vi "CRYMark Frame Above.vi"() -> ()   [LabVIEW 2013]
uses:
  <vilib>/Utility/miscctls.llb/LVPositionTypeDef.ctl
  SubVI/CRYMain Sub Window Global.vi
panel:
  in  "sMe":string
  in  "bShow":bool=TRUE
  in  "Above":bool
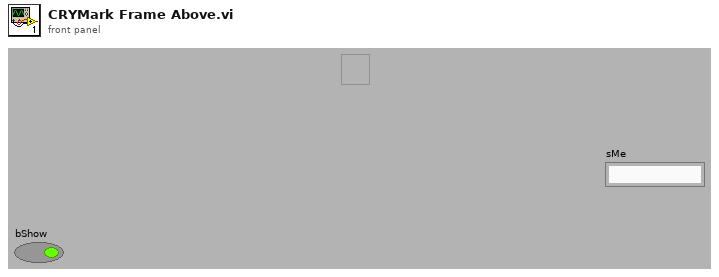
[diagram p1: front panel]
types:
  T1 = typedef "LVPositionTypeDef.ctl" = cluster{"Left":i32, "Top":i32}
  T2 = typedef "LVRectTypeDef.ctl" = cluster{"Left":i16, "Top":i16, "Right":i16, "Bottom":i16}
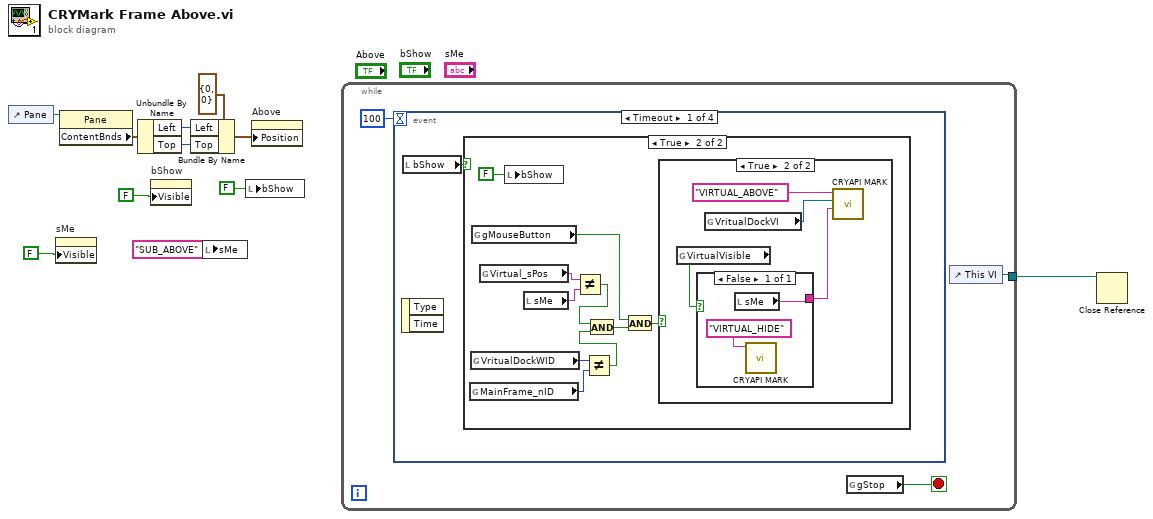
[diagram p0: block diagram]
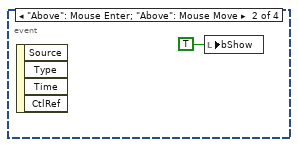
[diagram p4: hidden frame]
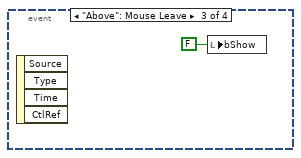
[diagram p5: hidden frame]
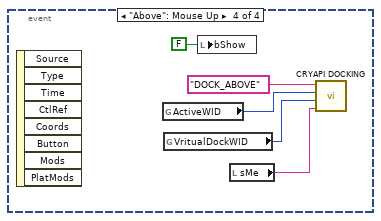
[diagram p6: hidden frame]
diagram:
  n1 = control-ref of="Pane"() -> (w11:refnum<vi>)
  n2 = property on="sMe" class="Str"("Visible"=FALSE) -> ()  [unwired: 2 in, 2 out]
  n3 = property class="Pane"(reference=w11) -> ("ContentBnds"=w10:T2)  [unwired: 1 in, 2 out]
  n4 = Unbundle By Name(w10) -> ("Left"=w9:i16, "Top"=w7:i16)
  n5 = property on="bShow" class="Bool (strict)"("Visible"=FALSE) -> ()  [unwired: 2 in, 2 out]
  n6 = Bundle By Name(cluster=T1 {"Left"=0, "Top"=0} ("Position"), "Left"=w9, "Top"=w7) -> (w6:T1)
  n7 = local write "sMe"("SUB_ABOVE" ("sMe")) -> ()
  n8 = local write "bShow"(FALSE ("bShow")) -> ()
  n9 = property on="Above" class="Bool (strict)"("Position"=w6) -> ()  [unwired: 2 in, 2 out]
  n10 = while {
    tunnel: [w12] -> w1
    stop <- w13 stop-if-true
    n11 = event shown="[0] Timeout" {
      selector: _ -> [_ _ _ _]
      dyn-events: _ -> [_ _ _ _]
      timeout: 100 -> [_ _ _ _]
      event Timeout {
        n12 = event-data() -> ()  [unwired: 3 out]
        n13 = local read "bShow"() -> (w15:bool)
        n14 = case shown="True" w15 {
          frame False {
          }
          frame True {
            n15 = global read "CRYMain Sub Window Global.vi" "MainFrame_nID"() -> (w24:i32)
            n16 = global read "CRYMain Sub Window Global.vi" "VritualDockWID"() -> (w23:i32)
            n17 = global read "CRYMain Sub Window Global.vi" "gMouseButton"() -> (w20:bool)
            n18 = global read "CRYMain Sub Window Global.vi" "Virtual_sPos"() -> (w19:string)
            n19 = local write "bShow"(FALSE ("bShow")) -> ()
            n20 = local read "sMe"() -> (w18:string)
            n21 = Not Equal?(x=w19, y=w18) -> (x != y?=w22:bool)
            n22 = Not Equal?(x=w23, y=w24) -> (x != y?=w16:bool)
            n23 = And(x=w22, y=w16) -> (x .and. y?=w21:bool)
            n24 = And(x=w20, y=w21) -> (x .and. y?=w25:bool)
            n25 = case shown="True" w25 {
              frame False {
              }
              frame True {
                n26 = global read "CRYMain Sub Window Global.vi" "VirtualVisible"() -> (w28:bool)
                n27 = case shown="False, True" w28 {
                  tunnel: [w30] -> w26
                  frame False {
                    n28 = local read "sMe"() -> (w30:string)
                    n29 = call "CRYAPI MARK.vi"("sAction"="VIRTUAL_HIDE") -> ()  [unwired: 3 in, 7 out]
                  }
                }
                n30 = global read "CRYMain Sub Window Global.vi" "VritualDockVI"() -> (w29:refnum<vi>)
                n31 = call "CRYAPI MARK.vi"("sAction"="VIRTUAL_ABOVE", "mVritual_VIRef"=w29, "sData"=w26) -> ()  [unwired: 1 in, 7 out]
              }
            }
          }
        }
      }
      event "Above": Mouse Enter; "Above": Mouse Move {
        n32 = event-data() -> ()  [unwired: 5 out]
        n33 = local write "bShow"(TRUE ("bShow")) -> ()
      }
      event "Above": Mouse Leave {
        n34 = event-data() -> ()  [unwired: 5 out]
        n35 = local write "bShow"(FALSE ("bShow")) -> ()
      }
      event "Above": Mouse Up {
        n36 = event-data() -> ()  [unwired: 9 out]
        n37 = global read "CRYMain Sub Window Global.vi" "ActiveWID"() -> (w37:i32)
        n38 = global read "CRYMain Sub Window Global.vi" "VritualDockWID"() -> (w35:i32)
        n39 = local write "bShow"(FALSE ("bShow")) -> ()
        n40 = local read "sMe"() -> (w34:string)
        n41 = call "CRYAPI DOCKING.vi"("sData"=w34, "nDWinID"=w35, "nSWinID"=w37, "sAction"="DOCK_ABOVE") -> ()  [unwired: 8 out]
      }
    }
    n42 = global read "CRYMain Sub Window Global.vi" "gStop"() -> (w13:bool)
    n43 = control-ref of="This VI"() -> (w12:refnum<vi>)
  }
  n44 = Close Reference(reference=w1) -> ()  [unwired: 1 in, 1 out]
